vi "Addon.Initialize.vi"(8 "error in (no error)":errorcluster, 10 "Diagnostics Basic Configuraiton":T2, 11 "Device Item Ref in":T1 format="%.0x") -> (0 "error out":errorcluster, 3 "Device Item Ref out":T1=18446744073709551615 format="%.0x")   [LabVIEW 2015, in "Diagnostics Addon System Explorer.lvlib"]
uses:
  Diagnostics Addon System Explorer.lvlib
  Types/Addon.Initialize.ctl
  Shared/Types/Protocol.ctl
  <vilib>/NI Veristand/Custom Device API/Custom Device Item Ref.ctl
  <vilib>/NI Veristand/Custom Device Tools/Custom Device Utility Library/NI VeriStand - Search for Item by Name.vi
  <vilib>/NI Veristand/Custom Device Tools/Custom Device Utility Library/NI VeriStand - Search for Item by GUID.vi
  Shared/SubVIs/Constants.vi
  Shared/Diagnostics Addon Shared.lvlib
  <vilib>/NI VeriStand/Custom Device Tools/Custom Device Utility Library/Custom Device Utility Library.lvlib
  <vilib>/NI/NI VeriStand Custom Device Import and Export Tool/ImportExport.lvlib
  <vilib>/NI VeriStand/Custom Device API/Custom Device API.lvlib
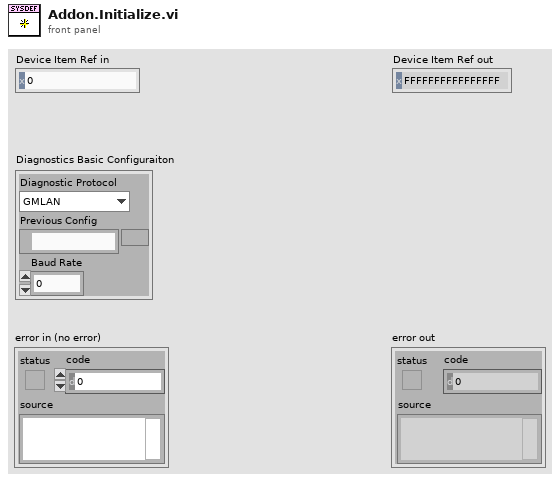
[diagram p1: front panel]
types:
  T1 = typedef "Custom Device API.lvlib/Custom Device Item Ref.ctl" = u64
  T2 = typedef "Diagnostics Addon System Explorer.lvlib/Addon.Initialize.ctl" = cluster{"Diagnostic Protocol":T3, "Previous Config":path, "Baud Rate":u32}
  T3 = typedef "Diagnostics Addon Shared.lvlib/Protocol.ctl" = enum16{"GMLAN", "KWP-2000", "UDS", "User-Defined"}
  T4 = typedef "Diagnostics Addon System Explorer.lvlib/SysDef.Export.ctl" = cluster{"Name":string, "Description":string, "Diagnostics Basic Configuraiton":T5, "DID Outputs":T9, "DID Inputs":T9, "PID Outputs":T9, "PID Inputs":T9, "DPIDs":T12, "DTC":T16, "NI 986x Support":T19, "Commands":T20, "Status":T21, "IO Controls":T22, "Routines":T25, "Memory Outputs":T9, "Memory Inputs":T9, "User Defined":T27}
  T5 = typedef "Diagnostics Addon Shared.lvlib/CAN.ctl" = cluster{"Interface":T6, "Baud Rate":u32, "Diagnostic Protocol":T3, "Transport Protocol":T7, "Transmit ID":u32, "Receive ID":u32, "Transmit Extension":u8, "Receive Extension":u8, "Receive UUDT ID":u32, "Enable Stream":bool, "VW TP Channel ID":u32, "Fill Frame":bool, "Fill Byte":u8, "Termination":bool, "LIN Cluster":refnum<k21>, "NAD":u8, "IO Mode":u32, "Max DLC":u16, "FD Baud Rate":u32, "Security":T8}
  T6 = typedef "Diagnostics Addon Shared.lvlib/CAN.Interface.ctl" = string
  T7 = typedef "Diagnostics Addon Shared.lvlib/Transport.ctl" = enum16{"ISO TP - Normal Mode", "ISO TP - Mixed Mode", "VW TP 2.0", "Diagnostics on IP", "ISO TP LIN"}
  T8 = typedef "Diagnostics Addon Shared.lvlib/Security.ctl" = cluster{"Source DLL Path":path, "Security Level":u8, "Target DLL Path":path}
  T9 = typedef "Diagnostics Addon System Explorer.lvlib/Frames.Export.ctl" = cluster{"Description":string, "Frames":T10[]}
  T10 = typedef "Diagnostics Addon System Explorer.lvlib/Frame.Export.ctl" = cluster{"Name":string, "Description":string, "ID":u32, "Signals":T11[]}
  T11 = typedef "Diagnostics Addon Shared.lvlib/Signal.ctl" = cluster{"Start Bit":u32, "Length":u32, "Scaling Factor":dbl, "Scaling Offset":dbl, "Minimum":dbl, "Maximum":dbl, "Data Type":u32, "Byte Order":u32, "Default Value":dbl, "Name":string, "Units":string, "Description":string}
  T12 = typedef "Diagnostics Addon System Explorer.lvlib/DPIDs.Export.ctl" = cluster{"Description":string, "DPIDs":T13[]}
  T13 = typedef "Diagnostics Addon System Explorer.lvlib/DPID.Export.ctl" = cluster{"Name":string, "Description":string, "DPID":T14}
  T14 = typedef "Diagnostics Addon Shared.lvlib/DPID.ctl" = cluster{"DPID ID":u8, "Speed":T15, "PIDs":u16[]}
  T15 = typedef "Diagnostics Addon Shared.lvlib/DPID.Rate.ctl" = enum16{"Slow", "Medium", "Fast"}
  T16 = typedef "Diagnostics Addon System Explorer.lvlib/DTC.Export.ctl" = cluster{"Description":string, "DTC descriptor":T17, "DTC Control":T18, "Created DTCs":u32}
  T17 = typedef "Diagnostics Addon Shared.lvlib/DTCDescriptor.ctl" = cluster{"DTC Byte Length":i32, "Status Byte Length":i32, "Add Data Byte Length":i32, "Byte Order":enum16{"Motorola", "Intel"}}
  T18 = typedef "Diagnostics Addon System Explorer.lvlib/DTCControl.Export.ctl" = cluster{"Description":string, "Signals":T11[]}
  T19 = typedef "Diagnostics Addon Shared.lvlib/986x.ctl" = cluster{"Enable":bool, "RIO Device":string, "Bitfile":path}
  T20 = typedef "Diagnostics Addon System Explorer.lvlib/Command.Export.ctl" = cluster{"Description":string}
  T21 = typedef "Diagnostics Addon System Explorer.lvlib/Status.Export.ctl" = cluster{"Description":string}
  T22 = typedef "Diagnostics Addon System Explorer.lvlib/IOControls.Export.ctl" = cluster{"Description":string, "IO Control Array":T23[]}
  T23 = typedef "Diagnostics Addon System Explorer.lvlib/IO.Export.ctl" = cluster{"Name":string, "Description":string, "ID":u16, "Signals":T24}
  T24 = typedef "Diagnostics Addon System Explorer.lvlib/CmdResp.Export.ctl" = cluster{"Cmd":T11[], "Response":T11[]}
  T25 = typedef "Diagnostics Addon System Explorer.lvlib/Routines.Export.ctl" = cluster{"Description":string, "Routine Array":T26[]}
  T26 = typedef "Diagnostics Addon System Explorer.lvlib/Routine.Export.ctl" = cluster{"Name":string, "Description":string, "ID":u16, "Start Parameters":T24, "Request Parameters":T24, "Stop Parameters":T24}
  T27 = typedef "Diagnostics Addon System Explorer.lvlib/UserDefined.Export.ctl" = cluster{"Description":string, "Groups":T28[]}
  T28 = typedef "Diagnostics Addon System Explorer.lvlib/UserDefined.Group.Export.ctl" = cluster{"Name":string, "Description":string, "Messages":T29[]}
  T29 = typedef "Diagnostics Addon System Explorer.lvlib/UserDefined.Group.Message.Export.ctl" = cluster{"Name":string, "Description":string, "Signals":T24}
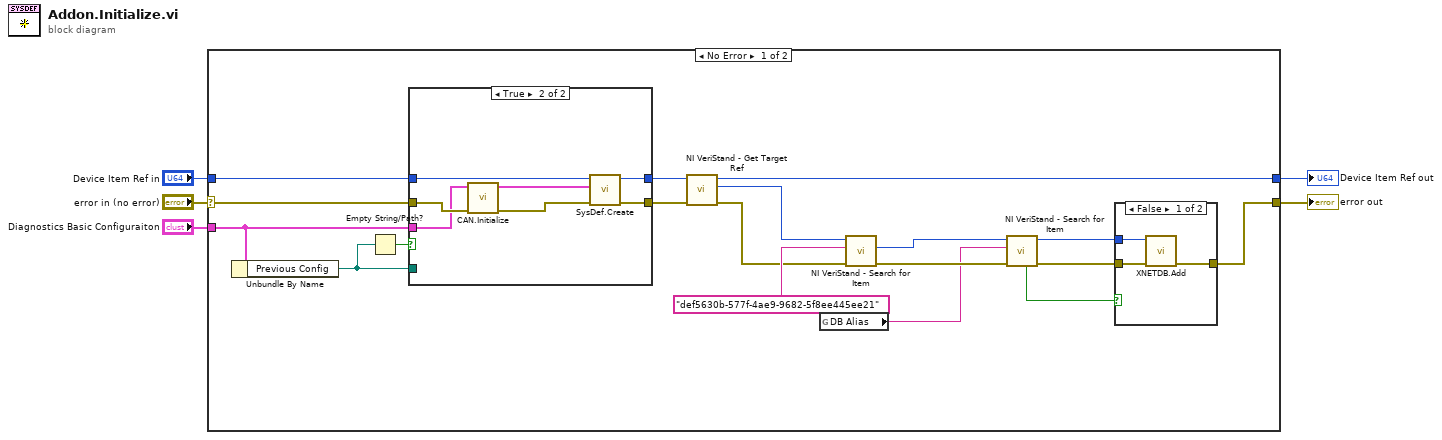
[diagram p0: block diagram]
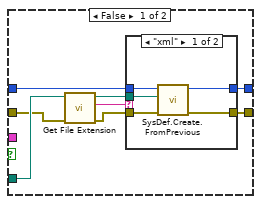
[diagram p3: hidden frame]
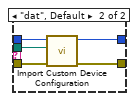
[diagram p4: hidden frame]
diagram:
  n1 = case shown="No Error" "error in (no error)" {
    selector: "error in (no error)" -> [w23 w53]
    tunnel: "Diagnostics Basic Configuraiton" -> [w21 _]
    tunnel: "Device Item Ref in" -> [w22 w54]
    tunnel: [w8 w54] -> w1
    tunnel: [w18 w53] -> w2
    frame No Error {
      n2 = Unbundle By Name(w21) -> ("Previous Config"=w19:path)
      n3 = Empty String/Path?(string/path=w19) -> (empty?=w20:bool)
      n4 = case shown="True" w20 {
        tunnel: [w35 w46] -> w10
        tunnel: [w34 w47] -> w13
        tunnel: w23 -> [w30 w52]
        tunnel: w22 -> [w33 w48]
        tunnel: w21 -> [_ w51]
        tunnel: w19 -> [w32 _]
        frame False {
          n5 = call <vilib>:"Get File Extension.vi"("error in (no error)"=w30, "file"=w32) -> ("error out"=w29:errorcluster, "lowercase file extension"=w28:string, "dup file"=w31:path)  [unwired: 5 in, 2 out]
          n6 = case shown="\"xml\"" w28 {
            tunnel: w29 -> [w37 w45]
            tunnel: [w39 w44] -> w35
            tunnel: [w38 w43] -> w34
            tunnel: w33 -> [w40 w42]
            tunnel: w31 -> [w36 w41]
            frame "xml" {
              n7 = call "SysDef.Create.FromPrevious.vi"("error in (no error)"=w37, "Path in"=w36, "Device Item Ref in"=w40) -> ("error out"=w38:errorcluster, "Ref out"=w39:T1)  [unwired: 7 in]
            }
            frame "dat", Default {
              n8 = call <vilib>:"Import Custom Device Configuration.vi"("error in (no error)"=w45, "Path"=w41, "NodeID"=w42) -> ("error out"=w43:errorcluster, "NodeID out"=w44:u64)  [unwired: 6 in, 1 out]
            }
          }
        }
        frame True {
          n9 = call "CAN.Initialize.vi"("error in (no error)"=w52, "Diagnostics Basic Configuraiton"=w51) -> ("error out"=w50:errorcluster, "Configuration"=w49:T4)  [unwired: 8 in]
          n10 = call "SysDef.Create.vi"("error in (no error)"=w50, "Configuration"=w49, "Device Item Ref in"=w48) -> ("error out"=w47:errorcluster, "Device Item Ref out"=w46:T1)  [unwired: 7 in]
        }
      }
      n11 = call <vilib>:"NI VeriStand - Get Target Ref.vi"("error in"=w13, "Item Ref in"=w10) -> ("error out"=w14:errorcluster, "Target Ref"=w12:T1, "Item Ref out"=w8:T1)  [unwired: 6 in, 1 out]
      n12 = global read "Constants.vi" "DB Alias"() -> (w11:string)
      n13 = call-poly <vilib>:"NI VeriStand - Search for Item.vi"("error in"=w14, "Item GUID"="def5630b-577f-4ae9-9682-5f8ee445ee21" ("string"), "Section Ref in"=w12) -> ("error out"=w15:errorcluster, "Item Ref"=w16:T1)  [unwired: 5 in, 2 out]
      n14 = call-poly <vilib>:"NI VeriStand - Search for Item.vi"("error in"=w15, "Item Name"=w11, "Section Ref in"=w16) -> ("error out"=w9:errorcluster, "Section Ref out"=w7:T1, "Found"=w6:bool)  [unwired: 5 in, 1 out]
      n15 = case shown="False" w6 {
        tunnel: [w26 w27] -> w18
        tunnel: w9 -> [w25 w27]
        tunnel: w7 -> [w24 _]
        frame False {
          n16 = call "XNETDB.Add.vi"("error in (no error)"=w25, "Databases Section Ref"=w24) -> ("error out"=w26:errorcluster)  [unwired: 9 in]
        }
        frame True {
        }
      }
    }
    frame Error {
    }
  }
  "error out" <- w2
  "Device Item Ref out" <- w1
